vi "GetProperties.vi"(8 "error in":errorcluster, 11 "WaveformChart in":refnum<class "WaveformChart.lvclass">) -> (0 "error out":errorcluster, 3 "WaveformChart out":refnum<class "WaveformChart.lvclass">)   [LabVIEW 2014, in "Raspberry Pi Compatible Compiler for LabVIEW.lvlib" / "WaveformChart.lvclass"]
uses:
  WaveformChart.lvclass
  WaveformChart.lvclass/WaveformChart.ctl
  GraphChart/GraphChart.lvclass
  Digital/Digital.lvclass
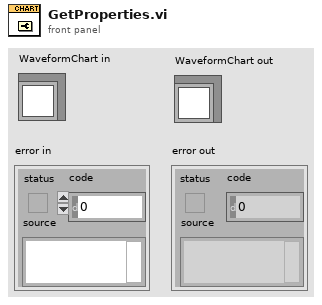
[diagram p1: front panel]
types:
  T1 = typedef "LVPositionTypeDef.ctl" = cluster{"Left":i32, "Top":i32}
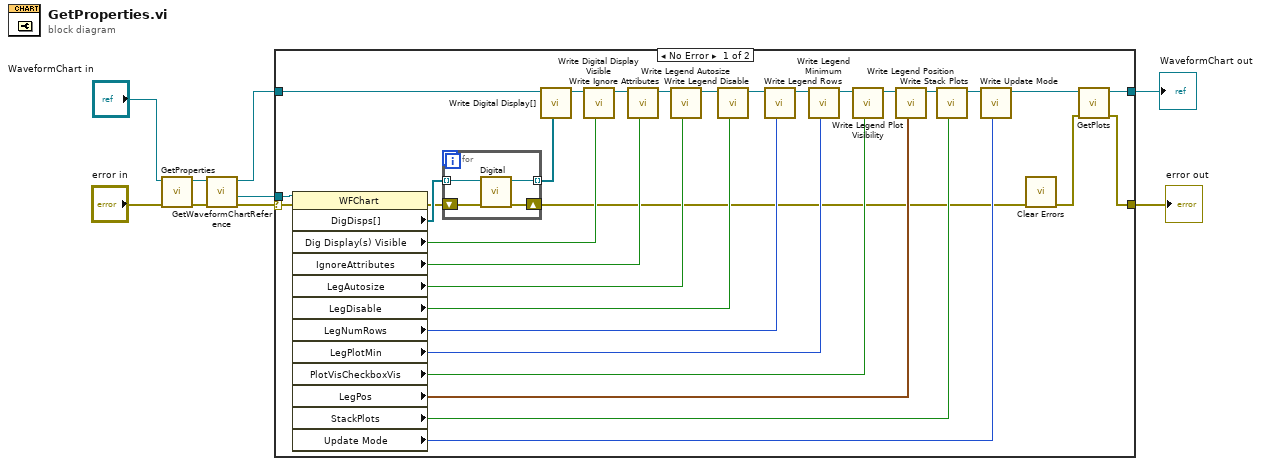
[diagram p0: block diagram]
diagram:
  n1 = call-parent "GetProperties.vi"("error in"="error in", "GraphChart in"="WaveformChart in") -> ("error out"=w6:errorcluster, "GraphChart out"=w7:refnum<class "WaveformChart.lvclass">)  [unwired: 8 in]
  n2 = call "GetWaveformChartReference.vi"("error in"=w6, "WFChart in"=w7) -> ("error out"=w5:errorcluster, "graph scale reference"=w4:refnum<vi>, "WFChart out"=w3:refnum<class "WaveformChart.lvclass">)  [unwired: 7 in]
  n3 = case shown="No Error" w5 {
    selector: w5 -> [w39 w45]
    tunnel: w4 -> [w40 _]
    tunnel: w3 -> [w34 w46]
    tunnel: [w12 w46] -> w2
    tunnel: [w10 w45] -> w1
    frame No Error {
      n4 = property class="WFChart"(reference=w40, error in=w39) -> (error out=w37:errorcluster, "DigDisps[]"=w38:refnum<vi>[], "Dig Display(s) Visible"=w35:bool, "IgnoreAttributes"=w26:bool, "LegAutosize"=w25:bool, "LegDisable"=w24:bool, "LegNumRows"=w22:u32, "LegPlotMin"=w21:u32, "PlotVisCheckboxVis"=w19:bool, "LegPos"=w18:T1, "StackPlots"=w17:bool, "Update Mode"=w16:u8)  [unwired: 1 out]
      n5 = for {
        tunnel: w38 -> [w43] mode=indexing
        shift-right: [w42] -> w15
        shift-left: w37 -> [w44]
        tunnel: [w41] -> w36 mode=indexing
        n6 = call "Digital.vi"("error in"=w44, "GObj Refnum"=w43) -> ("error out"=w42:errorcluster, "Digital out"=w41:refnum<class "Digital.lvclass">)  [unwired: 8 in]
      }
      n7 = call "Write Digital Display[].vi"("Digital Display[]"=w36, "WaveformChart in"=w34) -> ("WaveformChart out"=w33:refnum<class "WaveformChart.lvclass">)  [unwired: 7 in]
      n8 = call "Write Digital Display Visible.vi"("Digital Display Visible"=w35, "WaveformChart in"=w33) -> ("WaveformChart out"=w32:refnum<class "WaveformChart.lvclass">)  [unwired: 7 in]
      n9 = call "Write Ignore Attributes.vi"("Ignore Attributes"=w26, "WaveformChart in"=w32) -> ("WaveformChart out"=w31:refnum<class "WaveformChart.lvclass">)  [unwired: 7 in]
      n10 = call "Write Legend Autosize.vi"("Legend Autosize"=w25, "WaveformChart in"=w31) -> ("WaveformChart out"=w30:refnum<class "WaveformChart.lvclass">)  [unwired: 7 in]
      n11 = call "Write Legend Disable.vi"("Legend Disable"=w24, "WaveformChart in"=w30) -> ("WaveformChart out"=w23:refnum<class "WaveformChart.lvclass">)  [unwired: 7 in]
      n12 = call "Write Legend Rows.vi"("Legend Rows"=w22, "WaveformChart in"=w23) -> ("WaveformChart out"=w20:refnum<class "WaveformChart.lvclass">)  [unwired: 7 in]
      n13 = call "Write Legend Minimum.vi"("Legend Minimum"=w21, "WaveformChart in"=w20) -> ("WaveformChart out"=w29:refnum<class "WaveformChart.lvclass">)  [unwired: 7 in]
      n14 = call "Write Legend Plot Visibility.vi"("Legend Plot Visibility"=w19, "WaveformChart in"=w29) -> ("WaveformChart out"=w28:refnum<class "WaveformChart.lvclass">)  [unwired: 7 in]
      n15 = call "Write Legend Position.vi"("Legend Position"=w18, "WaveformChart in"=w28) -> ("WaveformChart out"=w14:refnum<class "WaveformChart.lvclass">)  [unwired: 7 in]
      n16 = call "Write Stack Plots.vi"("Stack Plots"=w17, "WaveformChart in"=w14) -> ("WaveformChart out"=w27:refnum<class "WaveformChart.lvclass">)  [unwired: 7 in]
      n17 = call "Write Update Mode.vi"("Update Mode"=w16, "WaveformChart in"=w27) -> ("WaveformChart out"=w13:refnum<class "WaveformChart.lvclass">)  [unwired: 7 in]
      n18 = call <vilib>:"Clear Errors.vi"("error in (no error)"=w15) -> ("error out"=w11:errorcluster)  [unwired: 5 in, 1 out]
      n19 = call "GetPlots.vi"("error in"=w11, "WaveformChart in"=w13) -> ("error out"=w10:errorcluster, "WaveformChart out"=w12:refnum<class "WaveformChart.lvclass">)  [unwired: 8 in]
    }
    frame Error {
    }
  }
  "error out" <- w1
  "WaveformChart out" <- w2
